vi "_WriteTopData_TDMS.vi"(10 "Top Data in":T1={"Status"={"id_sensor"=0, "Ind."=FALSE, "sample time"=0, "rov_states"=enum."INIT", "acquisition_time"=timestamp(0 s since 1904-01-01), "modo_ctrl"=enum."Manual"}, "DAQ"={"id_daq"=0, "id_sensor"=0, "gps_"={"lat"=0.0, "lon"=0.0, "alt"=0.0}, "usbl_"={"x"=0.0, "y"=0.0, "z"=0.0}, "vess_ahrs_"={"pitch"=0.0, "roll"=0.0, "yaw"=0.0}, "acquisition_time"=timestamp(0 s since 1904-01-01)}, "User Data"={"id_sensor"=0, "id_daq"=0, "ci_habilitada"=FALSE, "acquisition_time"=timestamp(0 s since 1904-01-01), "CI Data"={"joy_1x"=0.0, "joy_1y"=0.0, "joy_1z"=0.0, "joy_1thumb"=0.0, "joy_1botIzq"=0, "joy_1botder"=0, "joy_1gatillo"=0, "modo_1bot"=0, "modo_2bot"=0, "modo_3bot"=0, "modo_4bot"=0, "pot"=0.0, "enc"=0.0, "joy_2x"=0.0, "joy_2y"=0.0, "joy_2z"=0.0, "joy_2bot"=0, "botella_1bot"=0, "botella_2bot"=0, "botella_3bot"=0, "botella_4bot"=0, "corer_1bot"=0, "corer_2bot"=0, "a_in"=0.0, "dio1"=0, "dio2"=0, "dio3"=0, "ci_acc_x"=0.0, "ci_acc_y"=0.0, "ci_acc_z"=0.0}, "Surface Data"={"modo_1ind"=0, "modo_2ind"=0, "modo_3ind"=0, "modo_4ind"=0, "botella_1ind"=0, "botella_2ind"=0, "botella_3ind"=0, "botella_4ind"=0, "corer_1ind"=0, "corer_2ind"=0, "lars_vel"=0.0, "lars_fwd"=0, "lars_rev"=0}}, "Virtual CI"={"id_sensor"=0, "id_daq"=0, "bus_260v"=FALSE, "m_6"=FALSE, "m_5"=FALSE, "m_2"=FALSE, "m_1"=FALSE, "m_4"=FALSE, "m_3"=FALSE, "luz_1"=FALSE, "luz_2"=FALSE, "luz_3"=FALSE, "pot_m1"=0.0, "pot_m2"=0.0, "pot_m3"=0.0, "pot_m4"=0.0, "pot_m5"=0.0, "pot_m6"=0.0, "pot_l1"=0.0, "pot_l2"=0.0, "pot_l3"=0.0, "pot_gen"=0.0, "fuente_muestras"=FALSE, "bot_1"=FALSE, "bot_2"=FALSE, "bot_3"=FALSE, "bot_4"=FALSE, "corer_1"=FALSE, "corer_2"=FALSE, "pot_c1"=0.0, "pot_c2"=0.0, "virtual_ci"=FALSE, "acquisition_time"=timestamp(0 s since 1904-01-01)}, "Control"={"depth_PID"={"Kp"=0.0, "Ti"=0.03, "Td"=0.001}, "heading_PID"={"Kp"=0.05, "Ti"=0.03, "Td"=0.001}, "altitude_PID"={"Kp"=0.05, "Ti"=0.03, "Td"=0.001}, "depth_sp"=0.0, "heading_sp"=0.0, "altitude_sp"=0.0, "m_PID_en"=FALSE, "PID_reset"=FALSE, "acquisition_time"=timestamp(0 s since 1904-01-01), "motor_PID"={"Kp"=0.05, "Ti"=0.03, "Td"=0.001}, "m1_lo"=0.0, "m1_hi"=0.0, "m1_en"=TRUE, "m2_lo"=0.0, "m2_hi"=0.0, "m2_en"=TRUE, "m3_lo"=0.0, "m3_hi"=0.0, "m3_en"=TRUE, "m4_lo"=0.0, "m4_hi"=5.0, "m4_en"=TRUE, "m5_lo"=-5.0, "m5_hi"=5.0, "m5_en"=TRUE, "m6_lo"=-5.0, "m6_hi"=5.0, "m6_en"=TRUE, "modo_ctrl"=enum."Manual"}} {"Virtual CI"."pot_c2" step=0.1; "Virtual CI"."pot_c1" step=0.01; "Virtual CI"."pot_gen" step=1.0; "Virtual CI"."pot_l3" step=0.01; "Virtual CI"."pot_l2" step=0.01; "Virtual CI"."pot_l1" step=0.01; "Virtual CI"."pot_m6" step=0.01; "Virtual CI"."pot_m5" step=0.01; "Virtual CI"."pot_m4" step=0.01; "Virtual CI"."pot_m3" step=0.01; "Virtual CI"."pot_m2" step=0.01; "Virtual CI"."pot_m1" step=0.01; "DAQ"."vess_ahrs_"."yaw" format="%.2g"; "DAQ"."vess_ahrs_"."roll" format="%.2g"; "DAQ"."vess_ahrs_"."pitch" format="%.2g"; "DAQ"."usbl_"."z" format="%.7g"; "DAQ"."usbl_"."y" format="%.7g"; "DAQ"."usbl_"."x" format="%.7g"; "DAQ"."gps_"."alt" format="%.7g"; "DAQ"."gps_"."lon" format="%.7g"; "DAQ"."gps_"."lat" format="%.7g"}, 11 "Refnum in":refnum<k34>) -> (0 "error out":errorcluster, 3 "Refnum out":refnum<k34>)   [LabVIEW 2018]
uses:
  TypeDefsTopside/Top Data.ctl
  Shared/Type Defs/ROV States.ctl
  TypeDefsSubsea/Modos Control.ctl
  TypeDefsTopside/DAQ Top Data.ctl
  TypeDefsTopside/User Data.ctl
  TypeDefsTopside/CI Data.ctl
  TypeDefsTopside/Surface Input Data.ctl
  TypeDefsTopside/Virtual User Interface Data.ctl
  TypeDefsTopside/Top Control.ctl
  TypeDefsSubsea/Type Defs Subsea.lvlib
  TypeDefsTopside/Type Defs Topside.lvlib
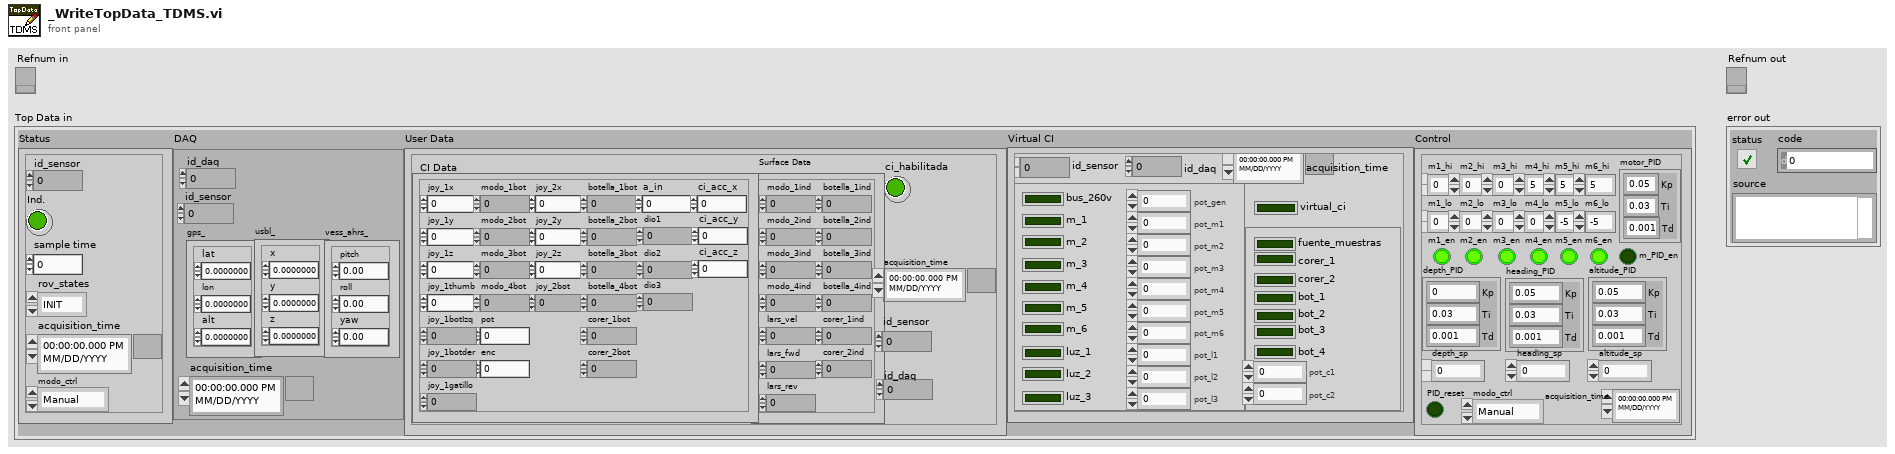
[diagram p1: front panel]
types:
  T1 = typedef "Type Defs Topside.lvlib/Top Data.ctl" = cluster{"Status":cluster{"id_sensor":u32, "Ind.":bool, "sample time":u32, "rov_states":T2, "acquisition_time":timestamp, "modo_ctrl":T3}, "DAQ":T4, "User Data":T5, "Virtual CI":T8, "Control":T9}
  T2 = typedef "Type Defs Subsea.lvlib/ROV States.ctl" = enum16{"INIT", "IDLE", "TEST", "RUN", "EMERGENCY", "EXIT"}
  T3 = typedef "Type Defs Subsea.lvlib/Modos Control.ctl" = enum16{"Manual", "Profundidad", "Altitud", "Rumbo", "P+R"}
  T4 = typedef "Type Defs Topside.lvlib/DAQ Top Data.ctl" = cluster{"id_daq":u32, "id_sensor":u32, "gps_":cluster{"lat":dbl, "lon":dbl, "alt":dbl}, "usbl_":cluster{"x":dbl, "y":dbl, "z":dbl}, "vess_ahrs_":cluster{"pitch":dbl, "roll":dbl, "yaw":dbl}, "acquisition_time":timestamp}
  T5 = typedef "Type Defs Topside.lvlib/User Data.ctl" = cluster{"id_sensor":u32, "id_daq":u64, "ci_habilitada":bool, "acquisition_time":timestamp, "CI Data":T6, "Surface Data":T7}
  T6 = typedef "Type Defs Topside.lvlib/CI Data.ctl" = cluster{"joy_1x":dbl, "joy_1y":dbl, "joy_1z":dbl, "joy_1thumb":dbl, "joy_1botIzq":u8, "joy_1botder":u8, "joy_1gatillo":u8, "modo_1bot":u8, "modo_2bot":u8, "modo_3bot":u8, "modo_4bot":u8, "pot":dbl, "enc":dbl, "joy_2x":dbl, "joy_2y":dbl, "joy_2z":dbl, "joy_2bot":u8, "botella_1bot":u8, "botella_2bot":u8, "botella_3bot":u8, "botella_4bot":u8, "corer_1bot":u8, "corer_2bot":u8, "a_in":dbl, "dio1":u8, "dio2":u8, "dio3":u8, "ci_acc_x":dbl, "ci_acc_y":dbl, "ci_acc_z":dbl}
  T7 = typedef "Type Defs Topside.lvlib/Surface Input Data.ctl" = cluster{"modo_1ind":u8, "modo_2ind":u8, "modo_3ind":u8, "modo_4ind":u8, "botella_1ind":u8, "botella_2ind":u8, "botella_3ind":u8, "botella_4ind":u8, "corer_1ind":u8, "corer_2ind":u8, "lars_vel":dbl, "lars_fwd":u8, "lars_rev":u8}
  T8 = typedef "Type Defs Topside.lvlib/Virtual User Interface Data.ctl" = cluster{"id_sensor":u32, "id_daq":u64, "bus_260v":bool, "m_6":bool, "m_5":bool, "m_2":bool, "m_1":bool, "m_4":bool, "m_3":bool, "luz_1":bool, "luz_2":bool, "luz_3":bool, "pot_m1":dbl, "pot_m2":dbl, "pot_m3":dbl, "pot_m4":dbl, "pot_m5":dbl, "pot_m6":dbl, "pot_l1":dbl, "pot_l2":dbl, "pot_l3":dbl, "pot_gen":dbl, "fuente_muestras":bool, "bot_1":bool, "bot_2":bool, "bot_3":bool, "bot_4":bool, "corer_1":bool, "corer_2":bool, "pot_c1":dbl, "pot_c2":dbl, "virtual_ci":bool, "acquisition_time":timestamp}
  T9 = typedef "Type Defs Topside.lvlib/Top Control.ctl" = cluster{"depth_PID":cluster{"Kp":dbl, "Ti":dbl, "Td":dbl}, "heading_PID":cluster{"Kp":dbl, "Ti":dbl, "Td":dbl}, "altitude_PID":cluster{"Kp":dbl, "Ti":dbl, "Td":dbl}, "depth_sp":dbl, "heading_sp":dbl, "altitude_sp":dbl, "m_PID_en":bool, "PID_reset":bool, "acquisition_time":timestamp, "motor_PID":cluster{"Kp":dbl, "Ti":dbl, "Td":dbl}, "m1_lo":dbl, "m1_hi":dbl, "m1_en":bool, "m2_lo":dbl, "m2_hi":dbl, "m2_en":bool, "m3_lo":dbl, "m3_hi":dbl, "m3_en":bool, "m4_lo":dbl, "m4_hi":dbl, "m4_en":bool, "m5_lo":dbl, "m5_hi":dbl, "m5_en":bool, "m6_lo":dbl, "m6_hi":dbl, "m6_en":bool, "modo_ctrl":T3}
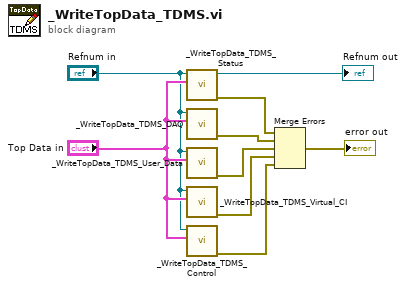
[diagram p0: block diagram]
diagram:
  n1 = call "_WriteTopData_TDMS_Status.vi"("Top Data in"="Top Data in", "Refnum in"="Refnum in") -> ("error out"=w6:errorcluster, "Refnum out"=→"Refnum out":refnum<k34>)  [unwired: 8 in]
  n2 = call "_WriteTopData_TDMS_DAQ.vi"("Top Data in"="Top Data in", "Refnum in"="Refnum in") -> ("error out"=w5:errorcluster)  [unwired: 8 in, 1 out]
  n3 = call "_WriteTopData_TDMS_User_Data.vi"("Top Data in"="Top Data in", "Refnum in"="Refnum in") -> ("error out"=w4:errorcluster)  [unwired: 8 in, 1 out]
  n4 = call "_WriteTopData_TDMS_Virtual_CI.vi"("Top Data in"="Top Data in", "Refnum in"="Refnum in") -> ("error out"=w3:errorcluster)  [unwired: 8 in, 1 out]
  n5 = call "_WriteTopData_TDMS_Control.vi"("Top Data in"="Top Data in", "Refnum in"="Refnum in") -> ("error out"=w2:errorcluster)  [unwired: 8 in, 1 out]
  n6 = Merge Errors(w6, w5, w4, w3, w2) -> (→"error out":errorcluster)
